vi "XY Graph Compute Multiplot Math Event.vi"(8 "Error In":errorcluster, 11 "Multiplot XY Graph":T1) -> (0 "Error Out":errorcluster, 1 "Message":string, 2 "Formula":string, 3 "Plot Name":string)   [LabVIEW 2021, in "XY Graph Add-Ons.lvlib"]
uses:
  XY Graph Add-Ons.lvlib
  XY Graph Refnum.ctl
  <vilib>/gmath/NI_Gmath.lvlib
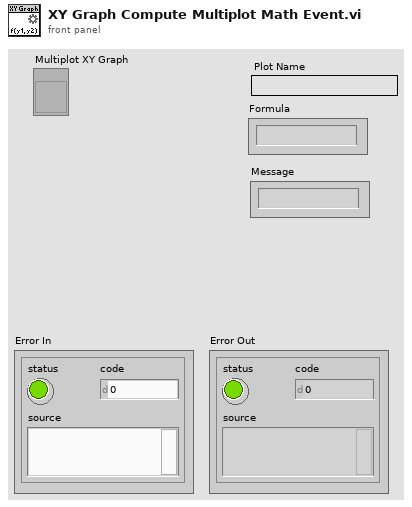
[diagram p1: front panel]
types:
  T1 = typedef "XY Graph Add-Ons.lvlib/XY Graph Refnum.ctl" = refnum<vi>
  T2 = typedef "Graphs.lvlib/Plot Destination.ctl" = enum32{"Plot 1", "Plot 2", "New Plot"}
  T3 = typedef "XY Graph Add-Ons.lvlib/XY Graph Plot Formula Definitiion.ctl" = cluster{"Plot 1 (y1)":u16, "Plot 2 (y2)":u16, "Plot Formula":string}
  T4 = typedef "XY Graph Add-Ons.lvlib/XY Plot Data.ctl" = cluster{"X Array":dbl[], "Y Array":dbl[]}
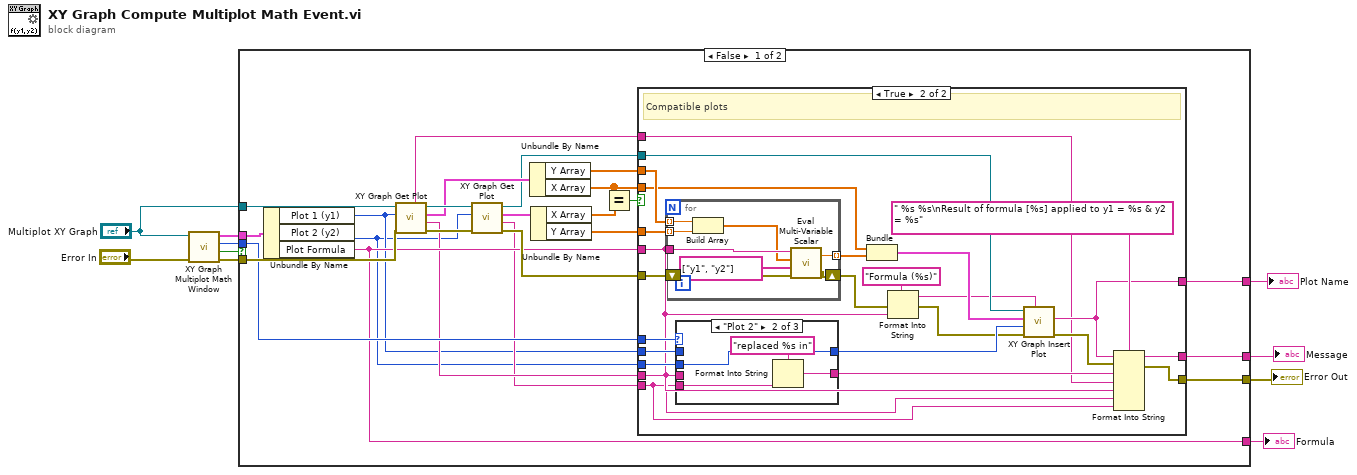
[diagram p0: block diagram]
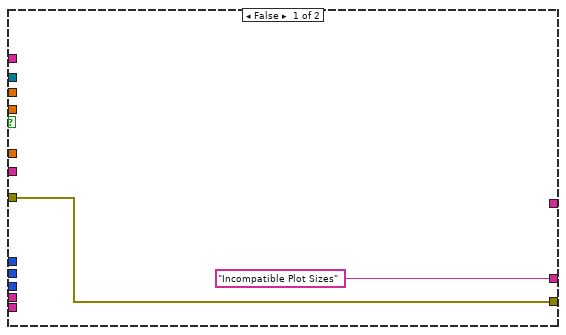
[diagram p2: hidden frame]
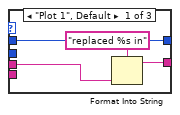
[diagram p3: hidden frame]
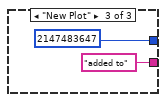
[diagram p4: hidden frame]
diagram:
  n1 = call "XY Graph Multiplot Math Window.vi"("Error In"="Error In", "XY Graph"="Multiplot XY Graph") -> ("Error Out"=w5:errorcluster, "Cancelled"=w6:bool, "Plot Destination Output"=w3:T2, "Plot Formula Definition output"=w4:T3)  [unwired: 6 in]
  n2 = case shown="False" w6 {
    tunnel: [w34 w80] -> w10
    tunnel: [w33 _] -> w9
    tunnel: [w32 _] -> w8
    tunnel: w5 -> [w26 w80]
    tunnel: w4 -> [w31 _]
    tunnel: w3 -> [w18 _]
    tunnel: "Multiplot XY Graph" -> [w27 _]
    tunnel: [w16 _] -> w1
    frame False {
      n3 = Unbundle By Name(w31) -> ("Plot 1 (y1)"=w12:u16, "Plot 2 (y2)"=w11:u16, "Plot Formula"=w16:string)
      n4 = call "XY Graph Get Plot.vi"("error in (no error)"=w26, "Plot Index (-1: last)"=w12, "XYGraph in"=w27) -> ("error out"=w19:errorcluster, "Plot Name"=w15:string, "Plot Data"=w25:T4, "XYGraph out"=w30:T1, "Graph Name"=w13:string)  [unwired: 4 in]
      n5 = call "XY Graph Get Plot.vi"("error in (no error)"=w19, "Plot Index (-1: last)"=w11, "XYGraph in"=w30) -> ("error out"=w20:errorcluster, "Plot Name"=w14:string, "Plot Data"=w29:T4, "XYGraph out"=w17:T1)  [unwired: 4 in, 1 out]
      n6 = Unbundle By Name(w25) -> ("Y Array"=w22:dbl[], "X Array"=w23:dbl[])
      n7 = Unbundle By Name(w29) -> ("X Array"=w28:dbl[], "Y Array"=w21:dbl[])
      n8 = Equal?(x=w23, y=w28) -> (x = y?=w24:bool)
      n9 = case shown="True" w24 {
        tunnel: [w35 w58] -> w34
        tunnel: ["Incompatible Plot Sizes" w59] -> w33
        tunnel: [_ w42] -> w32
        tunnel: w23 -> [_ w53]
        tunnel: w22 -> [_ w57]
        tunnel: w21 -> [_ w56]
        tunnel: w16 -> [_ w40]
        tunnel: w20 -> [w35 w55]
        tunnel: w18 -> [_ w48]
        tunnel: w12 -> [_ w47]
        tunnel: w11 -> [_ w45]
        tunnel: w17 -> [_ w51]
        tunnel: w15 -> [_ w39]
        tunnel: w14 -> [_ w38]
        tunnel: w13 -> [_ w37]
        frame False {
        }
        frame True {
          # "Compatible plots"
          n10 = for {
            tunnel: w57 -> [w79] mode=indexing
            tunnel: w56 -> [w78] mode=indexing
            tunnel: w40 -> [w76]
            tunnel: [w74] -> w54 mode=indexing
            shift-right: [w72] -> w52
            shift-left: w55 -> [w73]
            n11 = Build Array(w79, w78) -> (w75:dbl[])
            n12 = call <vilib>:"Eval Multi-Variable Scalar.vi"("error in (no error)"=w73, "Variables"=string[] ["y1", "y2"], "X Values"=w75, "formula"=w76) -> ("error out"=w72:errorcluster, "y value"=w74:dbl)
          }
          n13 = case shown="\"Plot 2\"" w48 {
            tunnel: w47 -> [w65 _ _]
            tunnel: [w65 w69 2147483647 ("Plot Index (Default Inf: Append to End)")] -> w46
            tunnel: w45 -> [_ w69 _]
            tunnel: [w64 w68 "added to" ("input 1")] -> w41
            tunnel: w39 -> [w62 _ _]
            tunnel: w38 -> [_ w66 _]
            frame "Plot 1", Default {
              n14 = Format Into String(format string="replaced %s in" ("input 1"), w62) -> (resulting string=w64:string)  [unwired: 2 in, 1 out]
            }
            frame "Plot 2" {
              n15 = Format Into String(format string="replaced %s in" ("input 1"), w66) -> (resulting string=w68:string)  [unwired: 2 in, 1 out]
            }
            frame "New Plot" {
            }
          }
          n16 = Bundle("X Array"=w53, w54) -> (w50:cluster{"X Array":dbl[], dbl[]})  [unwired: 1 in]
          n17 = Format Into String(format string="Formula (%s)" ("initial string"), error in=w52, w40) -> (resulting string=w49:string, error out=w44:errorcluster)  [unwired: 1 in]
          n18 = call "XY Graph Insert Plot.vi"("New Plot Name (Unchanged: \"\")"=w49, "Error In"=w44, "Plot Index (Default Inf: Append to End)"=w46, "New Plot"=w50, "Multiplot XY Graph Refnum in"=w51) -> ("Error Out"=w43:errorcluster, "Plot Name"=w42:string)  [unwired: 4 in, 1 out]
          n19 = Format Into String(format string=" %s %s\nResult of formula [%s] applied to y1 = %s & y2 = %s", initial string=w42, error in=w43, w41, w37, w40, w39, w38) -> (resulting string=w59:string, error out=w58:errorcluster)
        }
      }
    }
    frame True {
    }
  }
  "Error Out" <- w10
  "Formula" <- w1
  "Message" <- w9
  "Plot Name" <- w8
